vi "Read Non-Editable Rows.vi"(8 "error in (no error)":errorcluster, 11 "DataGrid in":refnum<class "DataGrid.lvclass">) -> (0 "error out":errorcluster, 2 "Non-Editable Rows":u32(colorbox), 3 "DataGrid out":refnum<class "DataGrid.lvclass">)   [LabVIEW 2017, in "DataGrid.lvclass"]
uses:
  DataGrid.lvclass
  DataGrid.lvclass/DataGrid.ctl
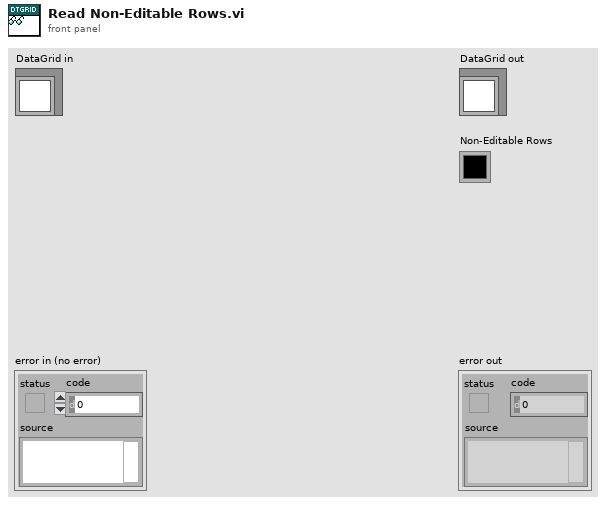
[diagram p1: front panel]
types:
  T1 = typedef "DataGrid.lvclass/State Data.ctl" = cluster{"Config":refnum<class "DataGrid Config.lvclass">, "Current Edit Position":T2, "Non-Editable Rows":u32, "Odd Rows":u32, "Even Rows":u32}
  T2 = typedef "LVRowAndColumnTypeDef.ctl" = cluster{"Row":i32, "Column":i32}
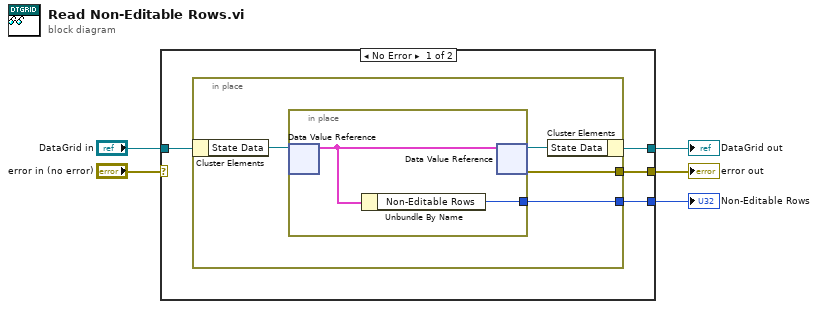
[diagram p0: block diagram]
diagram:
  n1 = case shown="No Error" "error in (no error)" {
    selector: "error in (no error)" -> [_ w16]
    tunnel: [w6 w16] -> w4
    tunnel: [w7 w17] -> w2
    tunnel: "DataGrid in" -> [w8 w17]
    tunnel: [w9 _] -> w1
    frame No Error {
      n2 = in-place {
        in-place-border: [w13] -> w9
        in-place-border: [w10] -> w6
        n3 = in-place-cluster #1(w8) -> ("State Data"=w12:refnum<data-value>)
        n4 = in-place {
          in-place-border: [w15] -> w13
          n5 = in-place-dvr #2(w12) -> (w14:T1)  [unwired: 1 out]
          n6 = Unbundle By Name(w14) -> ("Non-Editable Rows"=w15:u32)
          n7 = in-place-dvr #2(w14) -> (w11:refnum<data-value>, w10:errorcluster)
        }
        n8 = in-place-cluster #1("State Data"=w11) -> (w7:refnum<class "DataGrid.lvclass">)
      }
    }
    frame Error {
    }
  }
  "error out" <- w4
  "DataGrid out" <- w2
  "Non-Editable Rows" <- w1
